vi "Access SDO.vi"(8 "error in":errorcluster, 11 "OD Entry in":refnum<class "OD Entry.lvclass">) -> (0 "error out":errorcluster, 3 "OD Entry out":refnum<class "OD Entry.lvclass">)   [LabVIEW 2024, in "EDS.lvlib" / "OD Entry.lvclass"]
uses:
  OD Entry.lvclass
  OD Entry.lvclass/OD Entry.ctl
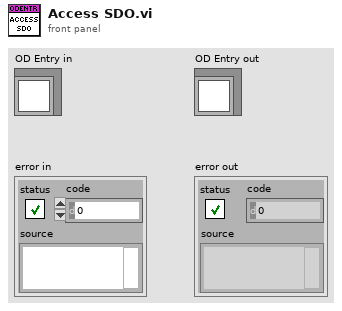
[diagram p1: front panel]
types:
  T1 = typedef "EDS.lvlib/Access Type.ctl" = enum16{"rw", "ro", "wo", "rwr", "rww", "@const", "UNKNOWN"}
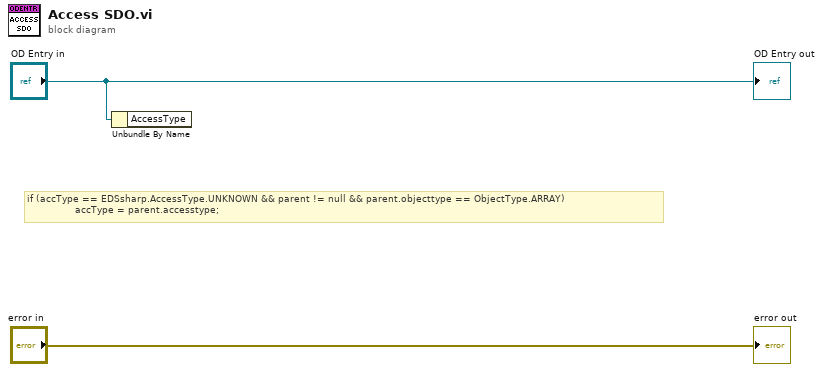
[diagram p0: block diagram]
diagram:
  # "if (accType == EDSsharp.AccessType.UNKNOWN && parent != null && parent.objecttype == ObjectType.ARRAY)\n                accType = parent.accesstype;"
  n1 = Unbundle By Name("OD Entry in") -> ("AccessType"=w1:T1)
  "error out" <- "error in"
  "OD Entry out" <- "OD Entry in"
